vi "Attenuator Calibrate.vi"(6 "Driver Refs":T1, 8 "error in (no error)":errorcluster, 11 "Current Calibration":T5) -> (0 "error out":errorcluster {"code" format="%.0x"}, 3 "Calibration Out":T5, 4 "Driver Refs Out":T1)   [LabVIEW 2011]
uses:
  TypeDefs/Attenuator Driver Refs.ctl
  drivers/ATT/ATT Driver Ref.ctl
  drivers/VNA/VNA Driver Ref.ctl
  drivers/SNA/SNA Driver Ref.ctl
  TypeDefs/Attenuator Calibration State.ctl
  drivers/VNA/VNA Command.ctl
  drivers/ATT/ATT Command.ctl
  TypeDefs/Attenuator Parameter to Measure.ctl
  S Parameter/TypeDefs/SP Parameter.ctl
  TypeDefs/Attenuator VNA Calibration State.ctl
  S Parameter/TypeDefs/SP Measurement Format.ctl
  TypeDefs/Attenuator ATT Stimulus.ctl
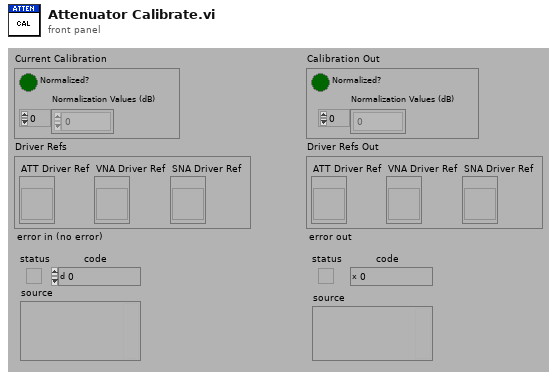
[diagram p1: front panel]
types:
  T1 = typedef "Attenuator Driver Refs.ctl" = cluster{"ATT Driver Ref":T2, "VNA Driver Ref":T3, "SNA Driver Ref":T4}
  T2 = typedef "ATT Driver Ref.ctl" = refnum<vi>
  T3 = typedef "VNA Driver Ref.ctl" = refnum<vi>
  T4 = typedef "SNA Driver Ref.ctl" = refnum<vi>
  T5 = typedef "Attenuator Calibration State.ctl" = cluster{"Normalized?":bool, "Normalization Values (dB)":dbl[]}
  T6 = typedef "Attenuator ATT Stimulus.ctl" = cluster{"Normalize":bool, "Value (dB)":dbl}
  T7 = typedef "Attenuator Parameter to Measure.ctl" = cluster{"Channel":i8, "Parameter":T8, "Calibration":T9, "Display Format":T10, "Pass?":bool}
  T8 = typedef "SP Parameter.ctl" = cluster{"Stimulus Port":i8, "Response Port":i8}
  T9 = typedef "Attenuator VNA Calibration State.ctl" = cluster{"State":bool, "String":string}
  T10 = typedef "SP Measurement Format.ctl" = enum32{"Log Mag", "Phase", "Delay", "Smith (R+jX)", "Polar (Re/Im)", "Linear Mag", "SWR", "Real", "Imaginary", "Smith (Lin/Phase)", "Smith (Log/Phase)", "Smith (Real/Imag)", "Smith (G+jB)", "Polar (Lin/Phase)", "Polar (Log/Phase)", "Expanded Phase", "Positive Phase", "Inverted Smith", "Unwrapped Phase", "Power Out", "Power In", "Linear Mag/Phase", "Log Mag/Phase", "Real/Imaginary"}
  T11 = typedef "ATT Command.ctl" = enum16{"LOAD", "INITIALIZE", "PRESET", "SET STIMULUS", "GET STIMULUS", "GET CALIBRATION", "CALIBRATE", "GET INFO", "RELEASE", "UNLOAD"}
  T12 = typedef "VNA Command.ctl" = enum16{"LOAD", "INITIALIZE", "PRESET", "GET STIMULUS", "SET STIMULUS", "GET CALIBRATION", "CALIBRATE", "RESTORE", "MEASURE", "RELEASE", "UNLOAD", "CONFIRM", "SORT"}
  T13 = typedef "SP Data.ctl" = cluster{"F0":dbl, "dF":dbl, "Data":cdb[][]}
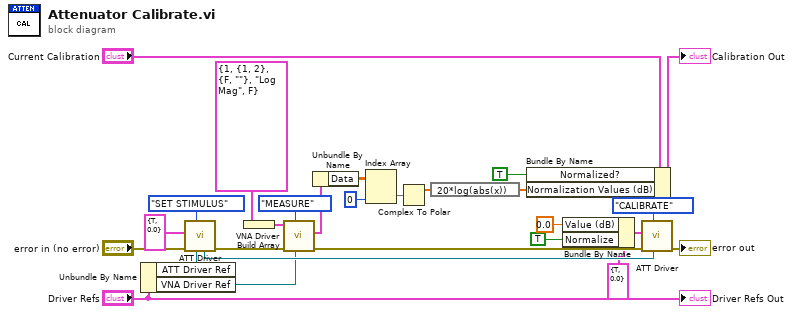
[diagram p0: block diagram]
diagram:
  n1 = Unbundle By Name("Driver Refs") -> ("ATT Driver Ref"=w9:T2, "VNA Driver Ref"=w10:T3)
  n2 = call "ATT Driver.vi"("Drv Refnum"=w9, "ATT Command"=ATT_Command."SET STIMULUS", "error in (no error)"="error in (no error)", "ATT Value In"=T6 {"Normalize"=TRUE, "Value (dB)"=0.0}) -> ("error out"=w20:errorcluster, "dup Drv Refnum"=w24:T2)  [unwired: 4 in, 2 out]
  n3 = Build Array(T7 {"Channel"=1, "Parameter"={"Stimulus Port"=1, "Response Port"=2}, "Calibration"={"State"=FALSE, "String"=""}, "Display Format"=enum."Log Mag", "Pass?"=FALSE} ("Parameter to Measure")) -> (w22:T7[])
  n4 = call "VNA Driver.vi"("Drv Refnum"=w10, "VNA Command"=VNA_Command."MEASURE", "error in (no error)"=w20, "Parameters to Measure"=w22) -> ("error out"=w14:errorcluster, "SP Data"=w19:T13)  [unwired: 3 in, 3 out]
  n5 = Unbundle By Name(w19) -> ("Data"=w17:cdb[][])
  n6 = Index Array(array=w17, index (col)=0 ("disabled index (col)")) -> (element=w15:cdb[])  [unwired: 1 in]
  n7 = Complex To Polar(r * e^(i*theta)=w15) -> (r=w18:dbl[])  [unwired: 1 out]
  n8 = expression code="20*log(abs(x))"(w18) -> (w3:dbl[])
  n9 = Bundle By Name(cluster="Current Calibration", "Normalized?"=TRUE, "Normalization Values (dB)"=w3) -> (→"Calibration Out":T5)
  n10 = Bundle By Name(cluster=T6 {"Normalize"=TRUE, "Value (dB)"=0.0} ("ATT Value In"), "Value (dB)"=0.0, "Normalize"=TRUE ("Normalized?")) -> (w12:T6)
  n11 = call "ATT Driver.vi"("Drv Refnum"=w24, "ATT Command"=ATT_Command."CALIBRATE", "error in (no error)"=w14, "ATT Value In"=w12) -> ("error out"=→"error out":errorcluster)  [unwired: 4 in, 3 out]
  "Driver Refs Out" <- "Driver Refs"
